vi "E709_Simple_Test.vi"() -> ()   [LabVIEW 2014, in "PiFOC.lvlib"]
doc: "This simple test VI is a stand-alone sample application. Use the \nHelp?Show Context Help menu sequence in the LabVIEW environment to display the Context Help window with the VI and control/indicator descriptions.\n\nSpecify \n¢ System no. (= 1 in a one-system configuration),\n¢ Interface (= RS232 or USB)\n¢ Timeout value (in milliseconds)\n¢ and interface settings first.\n\nThen start the VI. The VI will open a connection to the E-709 and query the controller for its identification string (*IDN?), the ID (SAI?) and stage name (CST?) of the connected axis and its current position value (POS?). The diagram shows how to combine the driver and support VIs for these tasks."
uses:
  PiFOC.lvlib
panel:
  in  "RS232 DaisyChain settings":T1={"Register DC"=FALSE, "DaisyChain Search?"=TRUE, "Device ID"=1}
  in  "Interface":u16(ring) items=["RS232", "USB", "RS232 DaisyChain"]
  out "Stage name":string[](array[string])
  in  "Wait":string="Please wait.\nChecking for correct baudrate."
  in  "USB settings":cluster{"S/N":string, "USB Search?":bool}={"S/N"="", "USB Search?"=TRUE}
  in  "RS232 settings":cluster{"Portnumber":i32, "Baudrate":u16}={"Portnumber"=0, "Baudrate"=4} {"Portnumber" items=["COM1", "COM2", "COM3", "COM4", "COM5", "COM6", "COM7", "COM8", "COM9", "COM10", "COM11", "COM12", "COM13", "COM14", "COM15", "COM16", "COM17", "COM18", "COM19", "COM20", "COM21", "COM22", "COM23", "COM24", "COM25", "COM26", "COM27", "COM28", "COM29", "COM30"]; "Baudrate" items=["9600", "14400", "19200", "38400", "57600", "115200"]}
  in  "error in":errorcluster
  in  "System no.":i32=1 min=1 step=1
  in  "Try different baudrates?":bool=TRUE
  in  "Timeout":i32=5000
  out "error out":errorcluster
  out "Position":dbl[](array[numeric]) format="%.6f"
  out "Conn. Axis":string[](array[string])
  out "Identification":string="\n"
  # "Simple E-709 communication test program"
  # "Select Interface settings first, then start the VI. If Interface = RS232 and you\ndon't know the correct Baudrate, leave \"Try different baudrates?\" TRUE. If\nInterface = USB and you don't know the serial number, leave \"USB Search?\" = TRUE. Then start the VI. \nThe VI will open the chosen port, query for connected axes (SAI?), position (POS?), stage name \n(CST?) and E-709 Identification (*IDN?). See VI and control/ indicator information for details."
  # "Only for\nInterface = \nRS232 or\nRS232 DaisyChain:"
  # "Only for\nInterface = \nRS232 or"
  # "Only for\nInterface = \nUSB:"
  # "Only for \nInterface =\nRS232 \nDaisyChain:"
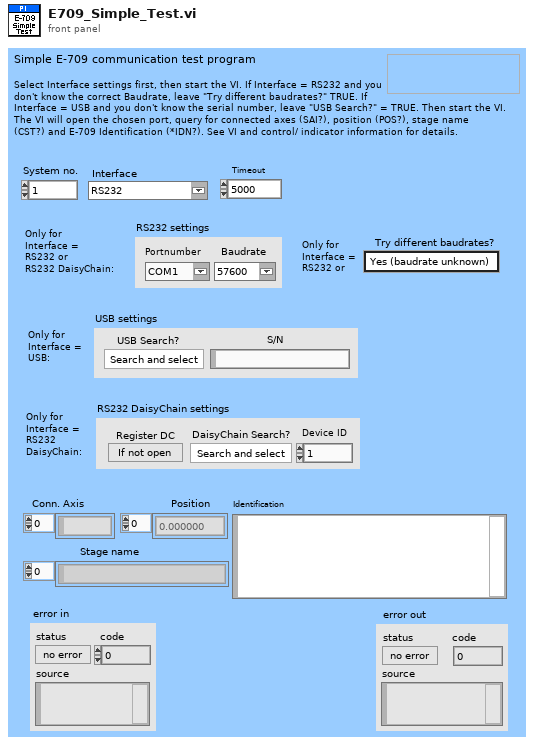
[diagram p1: front panel]
types:
  T1 = cluster{"Register DC":bool, "DaisyChain Search?":bool, "Device ID":i32}
  T2 = cluster{"input XON/XOFF":bool, "input HW Handshake":bool, "input alt HW HShk":bool, "output XON/XOFF":bool, "output HW Handshake":bool, "output alt HW HShk":bool, "XOFF byte":u8, "XON byte":u8, "parity error byte":u16}
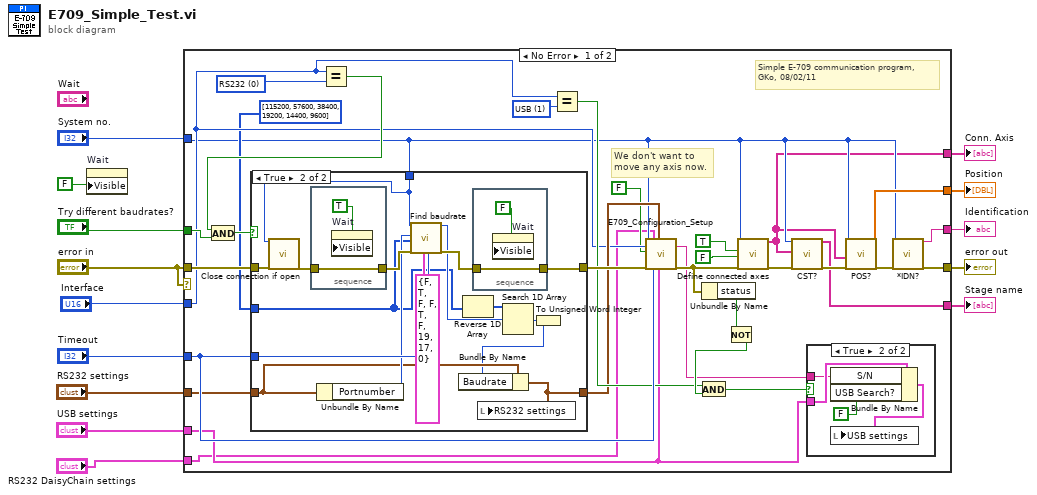
[diagram p0: block diagram]
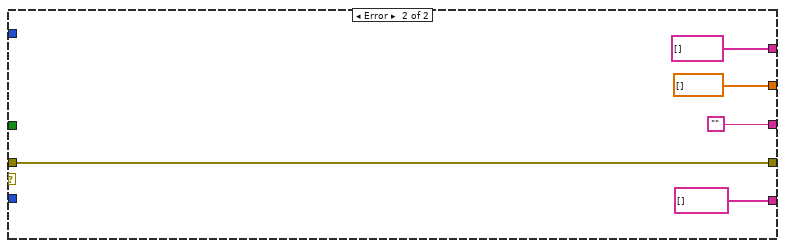
[diagram p4: hidden frame]
diagram:
  n1 = property on="Wait" class="Str"("Visible"=FALSE ("Write Attribute")) -> ()  [unwired: 2 in, 2 out]
  n2 = case shown="No Error" "error in" {
    tunnel: [w44 w77] -> w14
    tunnel: "error in" -> [w43 w77]
    tunnel: "System no." -> [w20 _]
    tunnel: "Try different baudrates?" -> [w31 _]
    tunnel: "Timeout" -> [w40 _]
    tunnel: [w39 "" ("Identification")] -> w8
    tunnel: [w38 dbl[] [] ("Num. values out")] -> w7
    tunnel: [w19 string[] [] ("Conn. Axes out")] -> w6
    tunnel: "Interface" -> [w24 _]
    tunnel: "USB settings" -> [w27 _]
    tunnel: "RS232 settings" -> [w26 _]
    tunnel: [w18 string[] [] ("Stage names")] -> w3
    tunnel: "RS232 DaisyChain settings" -> [w15 _]
    frame No Error {
      w29 = u16 1 items=["RS232", "USB"] ("Interface")
      w30 = u16 0 items=["RS232", "USB"] ("Interface")
      # "We don't want to\nmove any axis now."
      # "Simple E-709 communication program,\nGKo, 08/02/11"
      n3 = Equal?(x=w24, y=w30) -> (x = y?=w32:bool)
      n4 = And(x=w32, y=w31) -> (x .and. y?=w33:bool)
      n5 = case shown="True" w33 {
        tunnel: [w52 w68] -> w42
        tunnel: w43 -> [w52 w56]
        tunnel: w40 -> [_ w65]
        tunnel: w20 -> [_ w55]
        tunnel: u32[] [115200, 57600, 38400, 19200, 14400, 9600] ("Valid Baudrates") -> [_ w54]
        tunnel: w26 -> [w51 w61]
        tunnel: [w51 w59] -> w25
        frame False {
        }
        frame True {
          n6 = call "Close connection if open.vi"("System no."=w55, "error in"=w56) -> ("error out"=w57:errorcluster)  [unwired: 1 in, 16 out]
          n7 = stacked-sequence {
            tunnel: w57 -> [w70]
            tunnel: [w70] -> w66
            frame #0 {
              n8 = property on="Wait" class="Str"("Visible"=TRUE ("Write Attribute")) -> ()  [unwired: 2 in, 2 out]
            }
          }
          n9 = Unbundle By Name(w61) -> ("Portnumber"=w62:i32)
          n10 = call "Find baudrate.vi"("System no."=w55, "RS-232 Portnumber"=w62, "Valid Baudrates"=w54, "error in"=w66, "Flow control"=T2 {"input XON/XOFF"=FALSE, "input HW Handshake"=TRUE, "input alt HW HShk"=FALSE, "output XON/XOFF"=FALSE, "output HW Handshake"=TRUE, "output alt HW HShk"=FALSE, "XOFF byte"=19, "XON byte"=17, "parity error byte"=0}, "Timeout"=w65) -> ("Baudrate out"=w63:u32, "error out"=w67:errorcluster)  [unwired: 5 in, 7 out]
          n11 = Reverse 1D Array(array=w54) -> (reversed array=w53:u32[])
          n12 = stacked-sequence {
            tunnel: w67 -> [w71]
            tunnel: [w71] -> w68
            frame #0 {
              n13 = property on="Wait" class="Str"("Visible"=FALSE ("Write Attribute")) -> ()  [unwired: 2 in, 2 out]
            }
          }
          n14 = Search 1D Array(1D array=w53, element=w63) -> (index of element=w64:i32)  [unwired: 1 out]
          n15 = To Unsigned Word Integer(number=w64) -> (unsigned 16bit integer=w60:u16)
          n16 = Bundle By Name(cluster=w61, "Baudrate"=w60) -> (w59:cluster{"Portnumber":i32, "Baudrate":u16})
          n17 = local write "RS232 settings"(w59) -> ()
        }
      }
      n18 = Equal?(x=w24, y=w29) -> (x = y?=w28:bool)
      n19 = call "E709_Configuration_Setup.vi"("System no."=w20, "Interface"=w24, "Connected?"=FALSE, "error in"=w42, "RS232 DaisyChain settings"=w15, "Timeout"=w40, "RS232 settings"=w25, "USB settings"=w27) -> ("SN out"=w16:string, "error out"=w35:errorcluster)  [unwired: 6 in, 4 out]
      n20 = Unbundle By Name(w35) -> ("status"=w34:bool)
      n21 = Not(x=w34) -> (.not. x?=w36:bool)
      n22 = And(x=w28, y=w36) -> (x .and. y?=w37:bool)
      n23 = call "Define connected axes.vi"("System no."=w20, "Read from\ncontroller?"=TRUE ("Read from\nController"), "Invert\norder?"=FALSE ("Invert\nOrder"), "error in"=w35) -> ("Conn. Axes out"=w19:string[], "error out"=w22:errorcluster)  [unwired: 1 in, 13 out]
      n24 = call "CST?.vi"("System no."=w20, "Axes to query"=w19, "error in"=w22) -> ("Stage names"=w18:string[], "error out"=w21:errorcluster)  [unwired: 2 in, 13 out]
      n25 = case shown="True" w37 {
        tunnel: w27 -> [_ w50]
        tunnel: w16 -> [_ w49]
        frame False {
        }
        frame True {
          n26 = Bundle By Name(cluster=w50, "S/N"=w49, "USB Search?"=FALSE) -> (w47:cluster{"S/N":string, "USB Search?":bool})
          n27 = local write "USB settings"(w47) -> ()
        }
      }
      n28 = call "POS?.vi"("System no."=w20, "Axes to query"=w19, "error in"=w21) -> ("Position"=w38:dbl[], "error out"=w41:errorcluster)  [unwired: 3 in, 12 out]
      n29 = call "*IDN?.vi"("System no."=w20, "error in"=w41) -> ("Identification"=w39:string, "error out"=w44:errorcluster)  [unwired: 16 out]
    }
    frame Error {
    }
  }
  "error out" <- w14
  "Identification" <- w8
  "Position" <- w7
  "Conn. Axis" <- w6
  "Stage name" <- w3
